vi "Decimate (continuous).vi"   [LabVIEW 2017, in "NI_AALPro.lvlib"]
doc: "Continuously decimates the input sequence <B>X</B> by the <B>decimating factor</B> and the <B>averaging</B> Boolean control. Wire data to the <B>X</B> input to determine the polymorphic instance to use or manually select the instance."
uses:
  NI_AALPro.lvlib
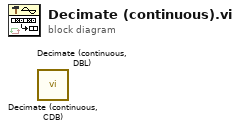
[diagram p0: block diagram]
diagram:
  n1 = call "Decimate (continuous, CDB).vi"() -> ()  [unwired: 10 in, 2 out]
  n2 = call "Decimate (continuous, DBL).vi"() -> ()  [unwired: 10 in, 2 out]
